vi "BB INV B Current Sense_v2.vi"(8 "error in (no error)":errorcluster, 11 "ControlBoard VISA":refnum<visa-resource-name>="ControlBoard") -> (0 "error out":errorcluster[](array[cluster]), 3 "Current Readings":dbl[](array[numeric]))   [LabVIEW 2022 SP3]
uses:
  ADCSelector BB.ctl
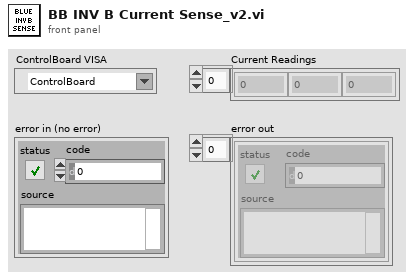
[diagram p1: front panel]
types:
  T1 = typedef "ADCSelector BB.ctl" = enum16{"INVA_ISENSE_U", "INVA_ISENSE_V", "INVA_ISENSE_W", "INVA_UDC", "INVA_TEMP", "HB_TEMP", "AUXB_TEMP", "VLINE_AB", "VLINE_BC", "VLINE_CA", "VSENSE_POS_24V", "VSENSE_POS_5V", "VSENSE_NEG_15V", "INVB_ISENSE_U", "INV_B_ISENSEV", "INVB_ISENSE_W", "INVB_UDC", "INVB_TEMP", "AUXA_TEMP", "AUXC_TEMP", "VOUT_AB", "VOUT_BC", "VOUT_CA", "VSENSE_POS_15V", "VSENSE_POS_3P3V", "TEST_POINT"}
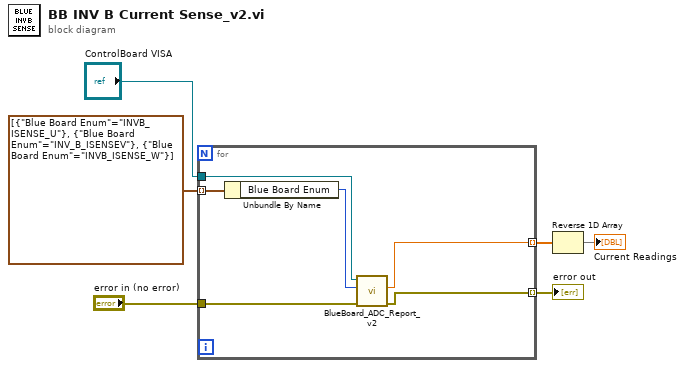
[diagram p0: block diagram]
diagram:
  n1 = for {
    tunnel: cluster{"Blue Board Enum":T1}[] [{"Blue Board Enum"=enum."INVB_ISENSE_U"}, {"Blue Board Enum"=enum."INV_B_ISENSEV"}, {"Blue Board Enum"=enum."INVB_ISENSE_W"}] -> [w10] mode=indexing
    tunnel: [w12] -> w6 mode=indexing
    tunnel: [w8] -> w5 mode=indexing
    tunnel: "error in (no error)" -> [w11]
    tunnel: "ControlBoard VISA" -> [w7]
    n2 = Unbundle By Name(w10) -> ("Blue Board Enum"=w9:T1)
    n3 = call "BlueBoard_ADC_Report_v2.vi"("error in (no error)"=w11, "Blue Board Enum"=w9, "ControlBoard VISA"=w7) -> ("error out"=w8:errorcluster, "Result"=w12:dbl)  [unwired: 5 in, 2 out]
  }
  "error out" <- w5
  n4 = Reverse 1D Array(array=w6) -> (reversed array=→"Current Readings":dbl[])
